vi "RESTful OutputMode To Text.vi"(1 "Output type":T1) -> (0 "Boolean Text":string)   [LabVIEW 2020]
uses:
  <vilib>/AppBuilder/AB_Classes/Source/RESTfulVI/Configure_RESTfulVI/AB_RESTful_OutputType.ctl
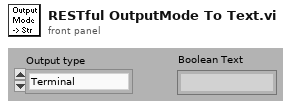
[diagram p1: front panel]
types:
  T1 = typedef "AB_RESTful_OutputType.ctl" = enum32{"Terminal", "Stream"}
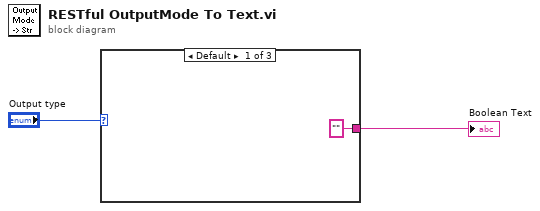
[diagram p0: block diagram]
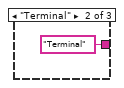
[diagram p2: hidden frame]
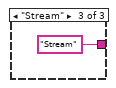
[diagram p3: hidden frame]
diagram:
  n1 = case shown="Default" "Output type" {
    tunnel: ["" ("Boolean Text") "Terminal" ("Boolean Text") "Stream" ("Boolean Text")] -> w2
    frame Default {
    }
    frame "Terminal" {
    }
    frame "Stream" {
    }
  }
  "Boolean Text" <- w2
